vi "Untitled 2.vi"() -> ()   [LabVIEW 2009]
panel:
  out "output 3":i32
  out "output 2":i32
  out "output 1":i32
  in  "input string":string
  out "remaining string":string
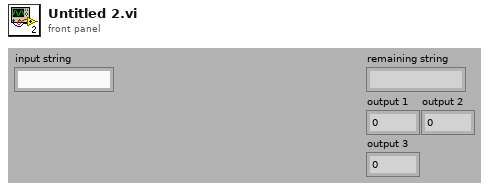
[diagram p1: front panel]
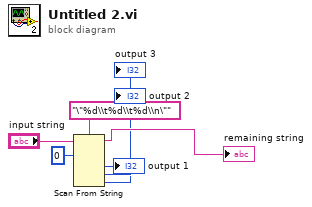
[diagram p0: block diagram]
diagram:
  n1 = Scan From String(format string="\"%d\\t%d\\t%d\\n\"", input string="input string", initial scan location=u32 0) -> (remaining string=→"remaining string":string, output 1=→"output 1":i32, output 2=→"output 2":i32, output 3=→"output 3":i32)  [unwired: 4 in, 2 out]
